vi "PH_Beckhoff_PPMA-Rods.evt call Warnlamp orange on.vi"(0 "i ref in":refnum<vi>, 2 "Instance name":string="N/A", 5 "error in":errorcluster) -> (14 "i ref out":refnum<vi>, 19 "error out":errorcluster)   [LabVIEW 2014, in "PH_Beckhoff_PPMA-Rods.lvlib"]
doc: "This VI calls an event by a simple call."
uses:
  PH_Beckhoff_PPMA-Rods.lvlib
  PH_Beckhoff_PPMA-Rods.Rods Tags.ctl
  PH_Beckhoff/PH_Beckhoff.lvlib
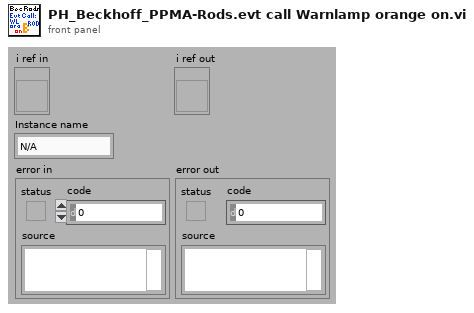
[diagram p1: front panel]
types:
  T1 = typedef "PH_Beckhoff_PPMA-Rods.lvlib/PH_Beckhoff_PPMA-Rods.Rods Tags.ctl" = enum16{"Rod-up", "earth-ok", "door-locked-K1", "door-locked-K2", "watervalve-closed", "Rods-Chain-A-up", "Rods-Chain-B-up", "HV-Warnlamp-orange", "HV-Warnlamp-green", "Status-Rods-PU-1", "Status-Rods-PU-2", "Status-Rods-PU-3", "Status-Rods-PU-4", "Status-Rods-PU-5", "Status-Rods-PU-6", "Status-Rods-PU-7", "Status-Rods-PU-8", "Status-Rods-PU-9", "Status-Rods-PU-10", "Status-Rods-FR", "Status-Rods-PILC"}
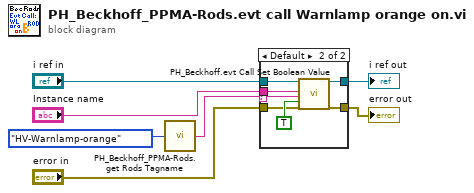
[diagram p0: block diagram]
diagram:
  n1 = call "PH_Beckhoff_PPMA-Rods.get Rods Tagname.vi"("Rods Tag"=PH_Beckhoff_PPMA-Rods.Rods_Tags."HV-Warnlamp-orange") -> ("Rods Tagname"=w2:string)
  n2 = case shown="Default" w2 {
    selector: w2 -> [_ w10]
    tunnel: [w8 w16] -> w7
    tunnel: "Instance name" -> [_ w14]
    tunnel: "error in" -> [w8 w13]
    tunnel: [w9 w12] -> w4
    tunnel: "i ref in" -> [w9 w11]
    frame "", "N/A" {
    }
    frame Default {
      n3 = call "PH_Beckhoff.evt Call Set Boolean Value.vi"("i ref in"=w11, "Beckhoff Instance"=w14, "Tagname to set"=w10, "Value"=TRUE ("NewVal"), "error in"=w13) -> ("i ref out"=w12:refnum<vi>, "error out"=w16:errorcluster)  [unwired: 13 in]
    }
  }
  "error out" <- w7
  "i ref out" <- w4
